vi "Replace4spaces.vi"(11 "String in":string) -> (2 "number of replacements":i32, 3 "String out":string)   [LabVIEW 2020]
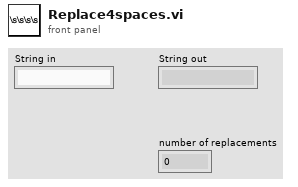
[diagram p1: front panel]
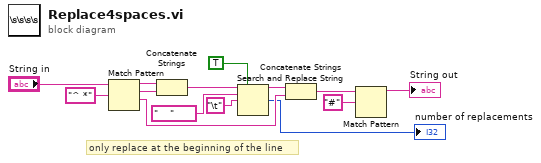
[diagram p0: block diagram]
diagram:
  # "only replace at the beginning of the line"
  n1 = Match Pattern(string="String in", regular expression="^ *" ("format string")) -> (before substring=w7:string, match substring=w8:string, after substring=w13:string)  [unwired: 1 in, 1 out]
  n2 = Concatenate Strings(w7, w8) -> (w9:string)
  n3 = Search and Replace String(replace all?=TRUE ("replace all? (F)"), input string=w9, search string="    " ("search"), replace string="\t" ("replace")) -> (result string=w12:string, number of replacements=→"number of replacements":i32)  [unwired: 4 in, 2 out]
  n4 = Concatenate Strings(w12, w13) -> (w14:string)
  n5 = Match Pattern(string=w14, regular expression="#") -> (before substring=→"String out":string)  [unwired: 1 in, 3 out]
